vi "Init_Test.vi"(8 "error in (no error)":errorcluster caption="entrée d'erreur (pas d'erreur)", 11 "Print_Label en entrée":refnum<class "Nodon_Send_Command_UART.lvclass">) -> (0 "error out":errorcluster caption="sortie d'erreur", 3 "Print_Label en sortie":refnum<class "Nodon_Send_Command_UART.lvclass">)   [LabVIEW 2020, in "Library Test.lvlib" / "Nodon_Send_Command_UART.lvclass"]
uses:
  Nodon_Send_Command_UART.lvclass
  C:/Users/ngarcin/OneDrive - Altyor/Standard TB/Class/Test/Test (Default)/Test (Default).lvclass
  Commun VI/TypeDef/Commande Test/Commande Value Type.ctl
  Commun VI/TypeDef/Commande Test/Commande Type Test.ctl
  Test_Wtih_Instr/Test_With_Inst.lvclass
  Instrument/Instrument (Default)/Class Instrument (Default).lvclass
  Nodon_Send_Command_UART.lvclass/Nodon_Send_Command_UART.ctl
  Commun VI/Library Commun.lvlib
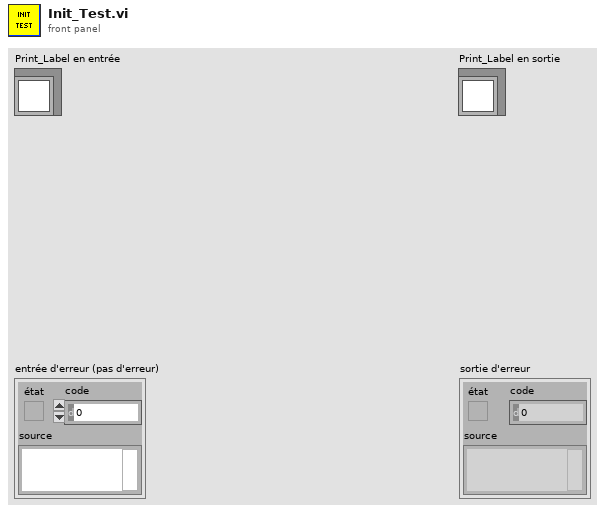
[diagram p1: front panel]
types:
  T1 = typedef "Library Commun.lvlib/Commande Type Test.ctl" = enum16{"Function", "Test", "Calculation"}
  T2 = typedef "Library Commun.lvlib/Commande Value Type.ctl" = enum16{"None", "String", "Number", "Timestamp", "Boolean", "Array"}
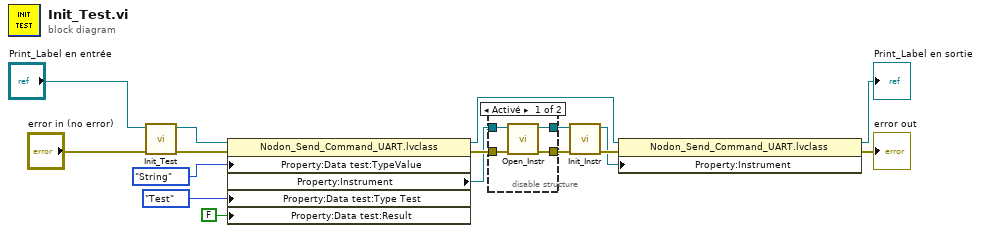
[diagram p0: block diagram]
diagram:
  n1 = call-parent "Init_Test.vi"("error in (no error)"="error in (no error)", "Test_With_Inst en entrée"="Print_Label en entrée") -> ("error out"=w13:errorcluster, "Test_With_Inst en sortie"=w14:refnum<class "Nodon_Send_Command_UART.lvclass">)  [unwired: 8 in]
  n2 = property class="Nodon_Send_Command_UART.lvclass"(reference=w14, error in=w13, "Property:Data test:TypeValue"=Commande_Value_Type."String" ("TypeValue"), "Property:Data test:Type Test"=Commande_Type_Test."Test" ("Type Test"), "Property:Data test:Result"=FALSE ("Result")) -> (reference out=w12:refnum<class "Nodon_Send_Command_UART.lvclass">, error out=w6:errorcluster, "Property:Instrument"=w3:refnum<class "Class Instrument (Default).lvclass">)
  n3 = disable-structure shown="Activé" {
    disable-tunnel: w6 -> [w20 w21]
    disable-tunnel: [w19 w21] -> w5
    disable-tunnel: w3 -> [w18 w22]
    disable-tunnel: [w17 w22] -> w2
    frame Enabled {
      n4 = call-dynamic "Open_Instr.vi"("error in (no error)"=w20, "Class Multimeter (Default) en entrée"=w18) -> ("error out"=w19:errorcluster, "Class Multimeter (Default) en sortie"=w17:refnum<class "Class Instrument (Default).lvclass">)  [unwired: 8 in]
    }
    frame Disabled {
    }
  }
  n5 = call-dynamic "Init_Instr.vi"("error in (no error)"=w5, "Class Instrument (Default) en entrée"=w2) -> ("error out"=w4:errorcluster, "Class Instrument (Default) en sortie"=w1:refnum<class "Class Instrument (Default).lvclass">)  [unwired: 8 in]
  n6 = property class="Nodon_Send_Command_UART.lvclass"(reference=w12, error in=w4, "Property:Instrument"=w1) -> (reference out=→"Print_Label en sortie":refnum<class "Nodon_Send_Command_UART.lvclass">, error out=→"error out":errorcluster)
